vi "chushihua.vi"(0 "单道1道宽":u16=3000, 1 "runtime(秒)":u16=10, 2 "单道1阈值":i32=100) -> ()   [LabVIEW 2014]
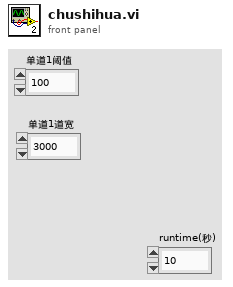
[diagram p1: front panel]
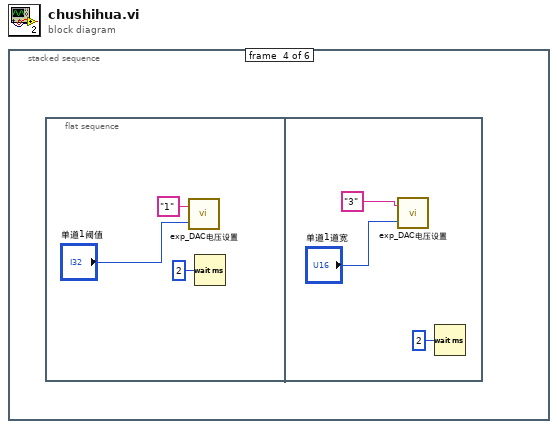
[diagram p0: block diagram]
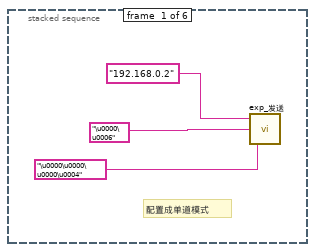
[diagram p2: hidden frame]
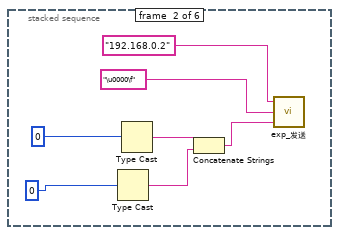
[diagram p3: hidden frame]
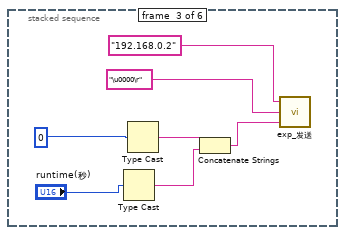
[diagram p4: hidden frame]
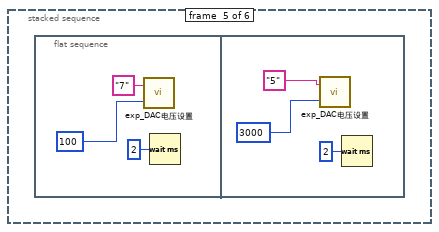
[diagram p5: hidden frame]
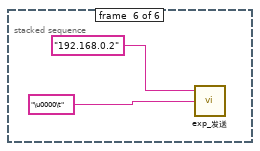
[diagram p6: hidden frame]
diagram:
  n1 = stacked-sequence {
    frame #0 {
      # "配置成单道模式"
      n2 = call "exp_发送.vi"("数据（32bit）"="\u0000\u0000\u0000\u0004", "命令(16bit)"="\u0000\u0006", "目标IP"="192.168.0.2") -> ()  [unwired: 1 out]
    }
    frame #1 {
      n3 = Type Cast(x=u16 0) -> (*(type *) &x=w6:string)  [unwired: 1 in]
      n4 = Type Cast(x=u16 0) -> (*(type *) &x=w7:string)  [unwired: 1 in]
      n5 = Concatenate Strings(w7, w6) -> (w8:string)
      n6 = call "exp_发送.vi"("数据（32bit）"=w8, "命令(16bit)"="\u0000\f", "目标IP"="192.168.0.2") -> ()  [unwired: 1 out]
    }
    frame #2 {
      n7 = Type Cast(x="runtime(秒)") -> (*(type *) &x=w13:string)  [unwired: 1 in]
      n8 = Type Cast(x=u16 0) -> (*(type *) &x=w14:string)  [unwired: 1 in]
      n9 = Concatenate Strings(w14, w13) -> (w15:string)
      n10 = call "exp_发送.vi"("数据（32bit）"=w15, "命令(16bit)"="\u0000\r", "目标IP"="192.168.0.2") -> ()  [unwired: 1 out]
    }
    frame #3 {
      n11 = flat-sequence {
        frame #0 {
          n12 = call "exp_DAC电压设置.vi"("电压"="单道1阈值", "cmd_channel(8bit)"="1") -> ()  [unwired: 1 in]
          n13 = Wait (ms)(milliseconds to wait=u32 2 ("等待时间（毫秒）")) -> ()  [unwired: 1 out]
        }
        frame #1 {
          n14 = call "exp_DAC电压设置.vi"("电压"="单道1道宽", "cmd_channel(8bit)"="3") -> ()  [unwired: 1 in]
          n15 = Wait (ms)(milliseconds to wait=u32 2 ("等待时间（毫秒）")) -> ()  [unwired: 1 out]
        }
      }
    }
    frame #4 {
      n16 = flat-sequence {
        frame #0 {
          n17 = call "exp_DAC电压设置.vi"("电压"=100, "cmd_channel(8bit)"="7") -> ()  [unwired: 1 in]
          n18 = Wait (ms)(milliseconds to wait=u32 2 ("等待时间（毫秒）")) -> ()  [unwired: 1 out]
        }
        frame #1 {
          n19 = call "exp_DAC电压设置.vi"("电压"=u16 3000, "cmd_channel(8bit)"="5") -> ()  [unwired: 1 in]
          n20 = Wait (ms)(milliseconds to wait=u32 2 ("等待时间（毫秒）")) -> ()  [unwired: 1 out]
        }
      }
    }
    frame #5 {
      n21 = call "exp_发送.vi"("命令(16bit)"="\u0000\t", "目标IP"="192.168.0.2") -> ()  [unwired: 1 in, 1 out]
    }
  }
